vi "Init Control.vi"(5 "Group":refnum<class "Group DBL.lvclass">, 6 "Period ms":i64, 7 "VolatusAPI":refnum<class "VolatusAPI.lvclass">, 8 "error in (no error)":errorcluster, 9 "Control MsgQ":refnum<class "MessageQ.lvclass">, 10 "Config Element":refnum<class "Config Element.lvclass">, 11 "SequencedValves in":refnum<class "SeqDelayControl.lvclass">) -> (0 "error out":errorcluster, 3 "SequencedValves out":refnum<class "SeqDelayControl.lvclass">)   [LabVIEW 2020, in "VolatusControl.lvlib" / "SeqDelayControl.lvclass"]
uses:
  SeqDelayControl.lvclass
  lv-cdm/CDM-Config/Config Element/Config Element.lvclass
  Volatus/VolatusAPI/VolatusAPI.lvclass
  Volatus/MessageQ/MessageQ.lvclass
  lv-vecto/Vecto/Group DBL/Group DBL.lvclass
  C:/dev/lv20CE/relink/lv-vecto/Vecto/Group/Group.lvclass
  SeqDelayControl.lvclass/SeqDelayControl.ctl
  lv-cdm/CDM-Config/Config Element/Owner.vi
  lv-cdm/CDM-Config/Config Manager/Lookup Descendant.vi
  lv-cdm/CDM-Config/Config Filter/Config Lookup.lvclass
  lv-vecto/Vecto/Group/Group.lvclass
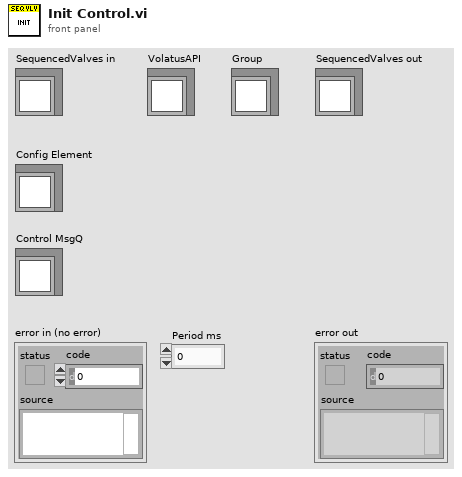
[diagram p1: front panel]
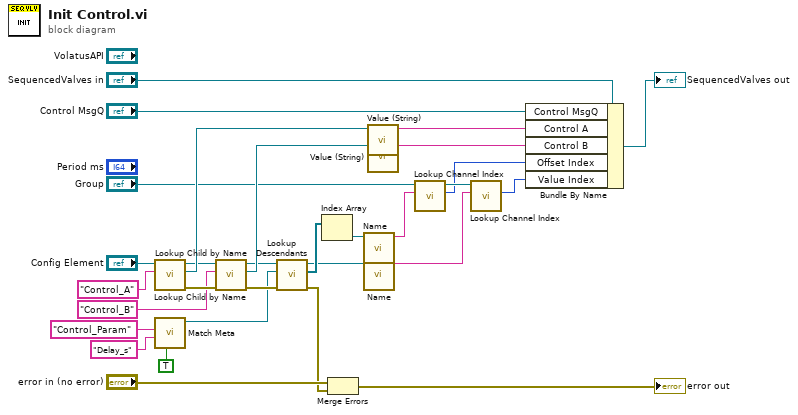
[diagram p0: block diagram]
diagram:
  n1 = call "Lookup Child by Name.vi"("Name"="Control_A", "Config Element in"="Config Element") -> ("error out"=w29:errorcluster, "Child"=w26:refnum<class "Config Element.lvclass">, "Config Element out"=w11:refnum<class "Config Element.lvclass">)  [unwired: 6 in, 1 out]
  n2 = call "Match Meta.vi"("Exact Value (F)"=TRUE, "Value (Any)"="Delay_s" ("Name"), "Name"="Control_Param") -> ("Config Lookup out"=w23:refnum<class "Config Lookup.lvclass">)  [unwired: 7 in, 1 out]
  n3 = call "Lookup Child by Name.vi"("error in (no error)"=w29, "Name"="Control_B", "Config Element in"=w11) -> ("error out"=w30:errorcluster, "Child"=w9:refnum<class "Config Element.lvclass">, "Config Element out"=w5:refnum<class "Config Element.lvclass">)  [unwired: 5 in, 1 out]
  n4 = call "Lookup Descendants.vi"("error in (no error)"=w30, "Lookup"=w23, "Config Element in"=w5) -> ("error out"=w1:errorcluster, "Descendants"=w22:refnum<class "Config Element.lvclass">[], "Config Element out"=w19:refnum<class "Config Element.lvclass">)  [unwired: 6 in]
  n5 = Index Array(array=w22) -> (element=w18:refnum<class "Config Element.lvclass">)  [unwired: 1 in]
  n6 = Merge Errors("error in (no error)", w1) -> (→"error out":errorcluster)
  n7 = call "Name.vi"("Config Element in"=w18) -> ("Name"=w17:string)  [unwired: 9 in, 1 out]
  n8 = call "Name.vi"("Config Element in"=w19) -> ("Name"=w15:string)  [unwired: 9 in, 1 out]
  n9 = call "Value (String).vi"("Config Element in"=w26) -> ("String Value"=w21:string)  [unwired: 9 in, 1 out]
  n10 = call "Value (String).vi"("Config Element in"=w9) -> ("String Value"=w10:string)  [unwired: 9 in, 1 out]
  n11 = call "Lookup Channel Index.vi"("Channel Name"=w17, "GroupAbstract in"="Group") -> ("Index"=w4:i32, "GroupAbstract out"=w16:refnum<class "Group DBL.lvclass">)  [unwired: 7 in, 1 out]
  n12 = call "Lookup Channel Index.vi"("Channel Name"=w15, "GroupAbstract in"=w16) -> ("Index"=w3:i32)  [unwired: 7 in, 2 out]
  n13 = Bundle By Name(cluster="SequencedValves in", "Control MsgQ"="Control MsgQ", "Control A"=w21, "Control B"=w10, "Offset Index"=w4, "Value Index"=w3) -> (→"SequencedValves out":refnum<class "SeqDelayControl.lvclass">)
